vi "UART Close.vi"(8 "Error In":errorcluster, 10 "UART Channel (0)":u8, 11 "LINX Resource":T1) -> (0 "Error Out":errorcluster, 3 "LINX Resource":T1)   [LabVIEW 2014, in "LMH-LINX.lvlib"]
doc: "Close the specified UART channel."
uses:
  <vilib>/MakerHub/LINX/LMH-LINX.lvlib
  <vilib>/MakerHub/LINX/Private/Type Defs/LINX Ref.ctl
  <vilib>/MakerHub/LINX/Private/Type Defs/Platform.ctl
  <vilib>/MakerHub/LINX/Private/Type Defs/Interface.ctl
  <vilib>/MakerHub/LINX/Private/Device/Type Defs/LINX Device Config.ctl
  <vilib>/MakerHub/LINX/Private/Device/Type Defs/TCP Config.ctl
  <vilib>/MakerHub/LINX/Private/Device/Type Defs/Channels.ctl
  <vilib>/MakerHub/LINX/Private/Type Defs/Peripheral.ctl
  <vilib>/MakerHub/LINX/Private/Utilties/Generate Error.vi
  <vilib>/MakerHub/LINX/Private/Local IO/Local IO.lvlib
  <vilib>/MakerHub/LINX/Private/Device/Device.lvlib
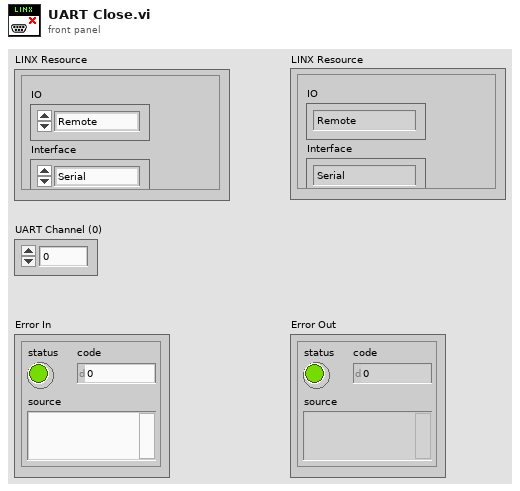
[diagram p1: front panel]
types:
  T1 = typedef "LMH-LINX.lvlib/LINX Ref.ctl" = cluster{"IO":T2, "Interface":T3, "LINX Device Config":T4}
  T2 = typedef "LMH-LINX.lvlib/Platform.ctl" = enum16{"Remote", "Local"}
  T3 = typedef "LMH-LINX.lvlib/Interface.ctl" = enum16{"Serial", "TCP"}
  T4 = typedef "LMH-LINX.lvlib/Device.lvlib/LINX Device Config.ctl" = cluster{"Interface":T3, "COM Port":refnum<visa-resource-name>, "TCP Configuration":T5, "Device Family":u8, "Device ID":u8, "Device Name":string, "TCP Ref":refnum<k5>, "Channels":T6}
  T5 = typedef "LMH-LINX.lvlib/Device.lvlib/TCP Config.ctl" = cluster{"IP Address":string, "Port":u16}
  T6 = typedef "LMH-LINX.lvlib/Channels.ctl" = cluster{"DI":u8[], "DO":u8[], "AI":u8[], "AO":u8[], "PWM":u8[], "QE":u8[], "UART":u8[], "I2C 2":u8[], "SPI":u8[], "CAN":u8[], "Servo":u8[], "AI Ref (V)":dbl, "AI Resolution (Bits)":u8, "AO Ref (V)":dbl, "AO Resolution (Bits)":u8}
  T7 = typedef "LMH-LINX.lvlib/Peripheral.ctl" = enum8{"DI", "DO", "AI", "AO", "PWM", "QE", "UART", "I2C", "SPI", "CAN", "Servo"}
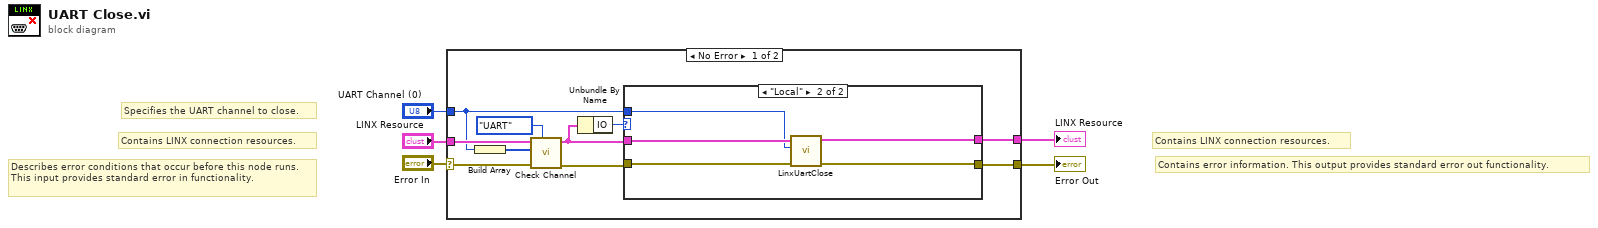
[diagram p0: block diagram]
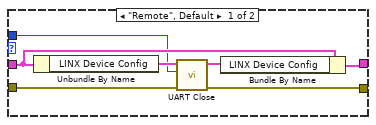
[diagram p2: hidden frame]
diagram:
  # "Specifies the UART channel to close."
  # "Contains LINX connection resources."
  # "Contains error information. This output provides standard error out functionality."
  # "Contains LINX connection resources."
  # "Describes error conditions that occur before this node runs. This input provides standard error in functionality."
  n1 = case shown="No Error" "Error In" {
    selector: "Error In" -> [w6 w29]
    tunnel: [w14 w29] -> w5
    tunnel: [w13 w28] -> w4
    tunnel: "LINX Resource" -> [w12 w28]
    tunnel: "UART Channel (0)" -> [w8 _]
    frame No Error {
      n2 = Build Array(w8) -> (w9:u8[])
      n3 = call <vilib>:"Check Channel.vi"("Peripheral"=Peripheral."UART", "Error In"=w6, "Channels"=w9, "LINX Resource"=w12) -> ("Error Out"=w10:errorcluster, "LINX Resource"=w11:T1)  [unwired: 5 in, 1 out]
      n4 = Unbundle By Name(w11) -> ("IO"=w15:T2)
      n5 = case shown="\"Local\"" w15 {
        tunnel: w10 -> [w18 w27]
        tunnel: w11 -> [w22 w25]
        tunnel: [w19 w26] -> w14
        tunnel: [w21 w23] -> w13
        tunnel: w8 -> [w16 w24]
        frame "Remote", Default {
          n6 = Unbundle By Name(w22) -> ("LINX Device Config"=w17:T4)
          n7 = call <vilib>:"UART Close.vi"("Error In"=w18, "UART Channel"=w16, "LINX Device Config"=w17) -> ("Error Out"=w19:errorcluster, "LINX Device Config"=w20:T4)  [unwired: 7 in]
          n8 = Bundle By Name(cluster=w22, "LINX Device Config"=w20) -> (w21:T1)
        }
        frame "Local" {
          n9 = call <vilib>:"LinxUartClose.vi"("Error In"=w27, "Uart Channel"=w24, "LINX Resource"=w25) -> ("Error Out"=w26:errorcluster, "LINX Resource"=w23:T1)  [unwired: 7 in]
        }
      }
    }
    frame Error {
    }
  }
  "Error Out" <- w5
  "LINX Resource" <- w4
